vi "Remove Named Filter.vi"(8 "error in (no error)":errorcluster, 10 "Filter Name":string, 11 "Main Display in":refnum<class "Main Display.lvclass">) -> (0 "error out":errorcluster, 3 "Main Display out":refnum<class "Main Display.lvclass">)   [LabVIEW 2016, in "Assert API Components.lvlib" / "Assert Display.lvlib" / "Main Display.lvlib" / "Main Display.lvclass"]
uses:
  Main Display.lvclass
  Main Display.lvclass/Main Display.ctl
  Assert API Components/Filter Configurations/Base Filter.lvclass/Base Filter.ctl
  Assert API Components/Filter Configurations/Base Filter.lvclass
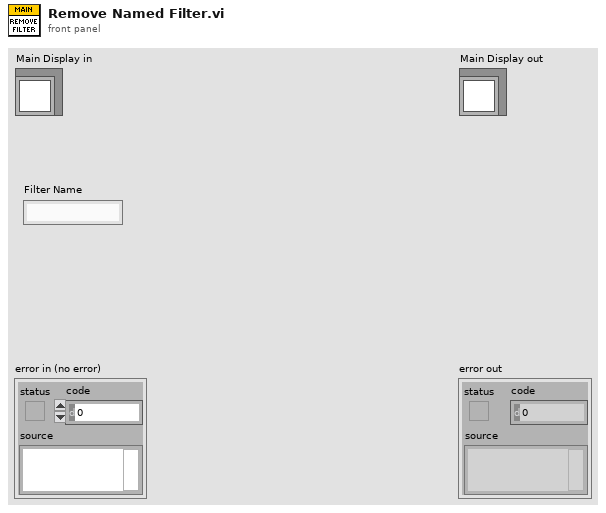
[diagram p1: front panel]
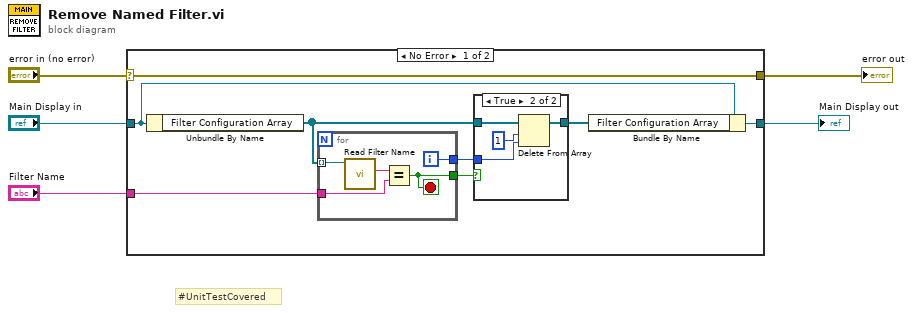
[diagram p0: block diagram]
diagram:
  # "#UnitTestCovered"
  n1 = case shown="No Error" "error in (no error)" {
    selector: "error in (no error)" -> [w13 w25]
    tunnel: [w13 w25] -> w4
    tunnel: [w7 w24] -> w2
    tunnel: "Main Display in" -> [w12 w24]
    tunnel: "Filter Name" -> [w11 _]
    frame No Error {
      n2 = Unbundle By Name(w12) -> ("Filter Configuration Array"=w9:refnum<class "Base Filter.lvclass">[])
      n3 = for {
        tunnel: w9 -> [w23] mode=indexing
        tunnel: w11 -> [w21]
        tunnel: [w20] -> w10
        tunnel: [w19] -> w8
        i -> [w19]
        stop <- w20 stop-if-true
        n4 = call "Read Filter Name.vi"("Base Filter in"=w23) -> ("Filter Name"=w22:string)  [unwired: 10 in]
        n5 = Equal?(x=w22, y=w21) -> (x = y?=w20:bool)
      }
      n6 = case shown="True" w10 {
        tunnel: w9 -> [w14 w18]
        tunnel: w8 -> [_ w16]
        tunnel: [w14 w15] -> w6
        frame False {
        }
        frame True {
          n7 = Delete From Array(array=w18, length=1, index=w16) -> (array with subset deleted=w15:refnum<class "Base Filter.lvclass">[])  [unwired: 1 out]
        }
      }
      n8 = Bundle By Name(cluster=w12, "Filter Configuration Array"=w6) -> (w7:refnum<class "Main Display.lvclass">)
    }
    frame Error {
    }
  }
  "error out" <- w4
  "Main Display out" <- w2
